vi "oa_Convert Triggered r0 to Index.vi"(9 "dr":dbl, 10 "r0":dbl, 11 "triggered r0":dbl) -> (0 "index":i32, 1 "dr out":dbl, 2 "r0 out":dbl)   [LabVIEW 2017, in "SoundVib_OAUtility.lvlib"]
uses:
  <vilib>/addons/Sound and Vibration/Order Analysis/Utility/SoundVib_OAUtility.lvlib
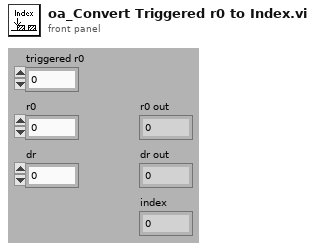
[diagram p1: front panel]
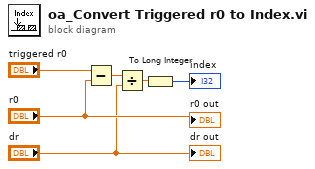
[diagram p0: block diagram]
diagram:
  n1 = Subtract(x="triggered r0", y="r0") -> (x-y=w5:dbl)
  n2 = Divide(x=w5, y="dr") -> (x/y=w6:dbl)
  n3 = To Long Integer(number=w6) -> (32bit integer=→"index":i32)
  "dr out" <- "dr"
  "r0 out" <- "r0"
